vi "Close.vi"(8 "error in (no error)":errorcluster, 11 "Motor-GWInstek in":refnum<class "Motor-GWInstek.lvclass">) -> (0 "error out":errorcluster, 3 "Motor-GWInstek out":refnum<class "Motor-GWInstek.lvclass">)   [LabVIEW 2013, in "PowderDeposition.lvlib" / "Motor-GWInstek.lvclass"]
uses:
  Motor-GWInstek.lvclass
  <instrlib>/GPD-2303/GPD-2303.lvlib
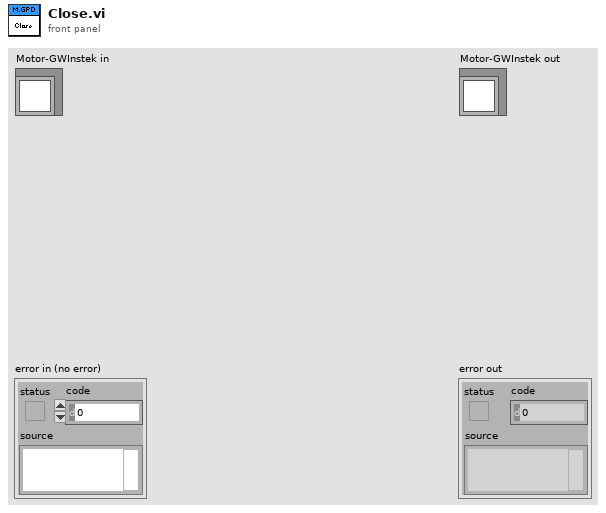
[diagram p1: front panel]
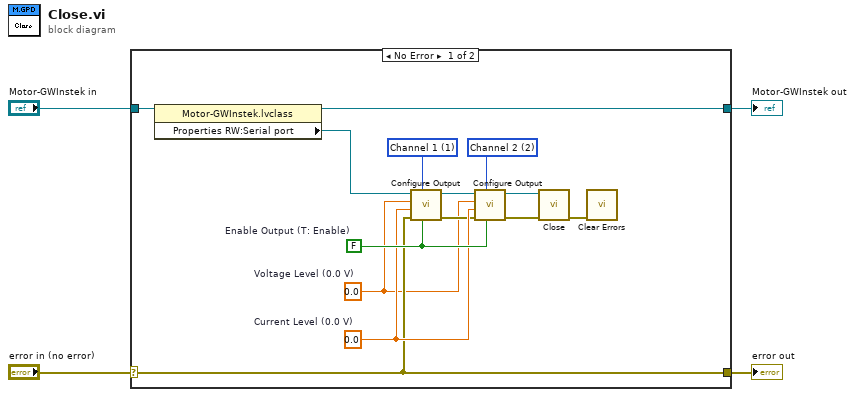
[diagram p0: block diagram]
diagram:
  n1 = case shown="No Error" "error in (no error)" {
    selector: "error in (no error)" -> [w8 w20]
    tunnel: [w8 w20] -> w3
    tunnel: [w16 w19] -> w1
    tunnel: "Motor-GWInstek in" -> [w17 w19]
    frame No Error {
      w9 = 0.0  # Current Level (0.0 V)
      w5 = 0.0  # Voltage Level (0.0 V)
      w10 = FALSE  # Enable Output (T: Enable)
      w11 = 1 items=["Channel 1"=1, "Channel 2"=2] ("Channel (1: Channel 1)")
      w12 = 2 items=["Channel 1"=1, "Channel 2"=2] ("Channel (1: Channel 1)")
      n2 = property class="Motor-GWInstek.lvclass"(reference=w17) -> (reference out=w16:refnum<class "Motor-GWInstek.lvclass">, "Properties RW:Serial port"=w15:refnum<visa-resource-name>)  [unwired: 1 in, 1 out]
      n3 = call <instrlib>:"Configure Output.vi"("Enable Output (T: Enable)"=w10, "Channel (1: Channel 1)"=w11, "error in (no error)"=w8, "Current Level (0.0 V)"=w9, "Voltage Level (0.0 V)"=w5, "VISA resource name"=w15) -> ("error out"=w7:errorcluster, "VISA resource name out"=w14:refnum<visa-resource-name>)  [unwired: 4 in]
      n4 = call <instrlib>:"Configure Output.vi"("Enable Output (T: Enable)"=w10, "Channel (1: Channel 1)"=w12, "error in (no error)"=w7, "Current Level (0.0 V)"=w9, "Voltage Level (0.0 V)"=w5, "VISA resource name"=w14) -> ("error out"=w6:errorcluster, "VISA resource name out"=w13:refnum<visa-resource-name>)  [unwired: 4 in]
      n5 = call <instrlib>:"Close.vi"("error in (no error)"=w6, "VISA resource name"=w13) -> ("error out"=w18:errorcluster)  [unwired: 9 in]
      n6 = call <vilib>:"Clear Errors.vi"("error in (no error)"=w18) -> ()  [unwired: 6 in, 1 out]
    }
    frame Error {
    }
  }
  "error out" <- w3
  "Motor-GWInstek out" <- w1
